vi "BotSpeak.Com.vi"(1 "To Send":string, 2 "Connection In":T1) -> (3 "error out":errorcluster, 4 "Sent":string, 5 "Reply":string, 6 "Connection out":T1)   [LabVIEW 2012]
uses:
  <userlib>/BotSpeak/VIs/SubVIs/CommState.ctl
  <userlib>/BotSpeak/VIs/Direct/BotSpeak_Control.ctl
  <userlib>/BotSpeak/VIs/SubVIs/BotSpeak_Globals.vi
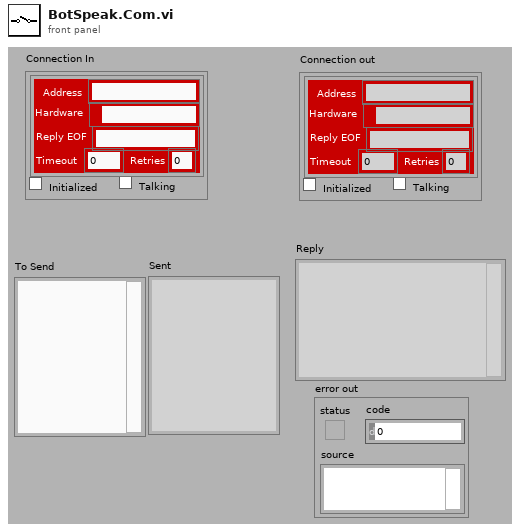
[diagram p1: front panel]
types:
  T1 = typedef "CommState.ctl" = cluster{"Bot Settings":T2, "Initialized":bool, "Talking":bool}
  T2 = typedef "BotSpeak_Control.ctl" = cluster{"Address":string, "Reply EOF":string, "Hardware":path, "Retries":i8, "Timeout":i32}
  T3 = typedef "BotSpeak.HardwareSpecs.ctl" = cluster{"Hardware Name":string, "Hardware URL":string, "ComType":enum16{"Undefined", "Serial", "TCPIP", "Console"}, "TCP Port":i32, "DefaultAddress":string, "Retries":i32, "Translate":enum16{"None", "Tiny", "URAPI"}, "MaxScriptSize":i32, "MaxVarNumber":i32, "StartupWait":i32, "Patience":i32, "Startup Patience":i32, "Hardware Help":string, "Com Protocol":string, "Translator":cluster{"BotSpeak CMD":string, "CMD out":string}[], "Init Code":string, "Variable Format":enum16{"INT", "FLOAT", "FIXED"}}
  T4 = cluster{"BotSpeak CMD":string, "CMD out":string}[]
  T5 = enum16{"Undefined", "Serial", "TCPIP", "Console"}
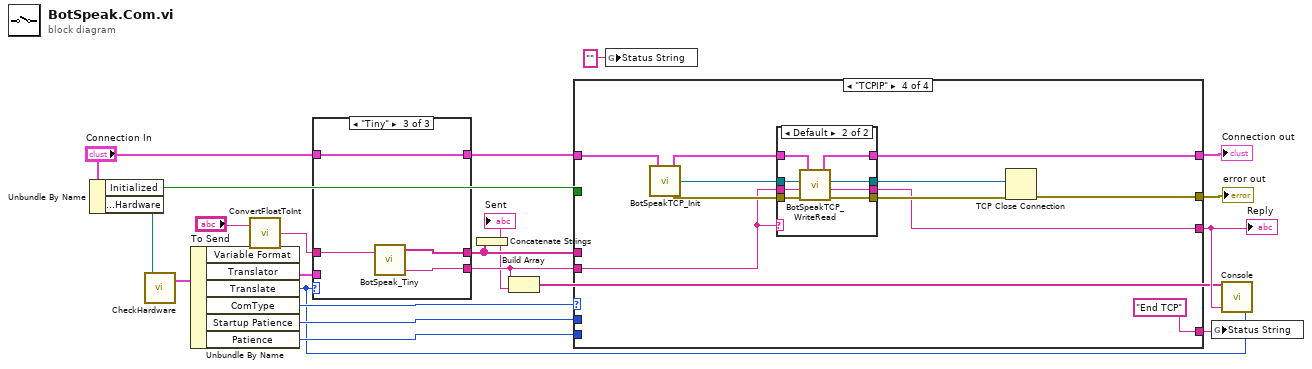
[diagram p0: block diagram]
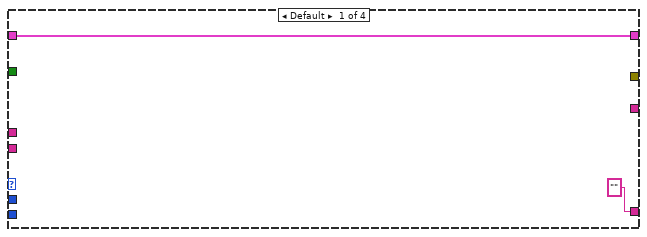
[diagram p2: hidden frame]
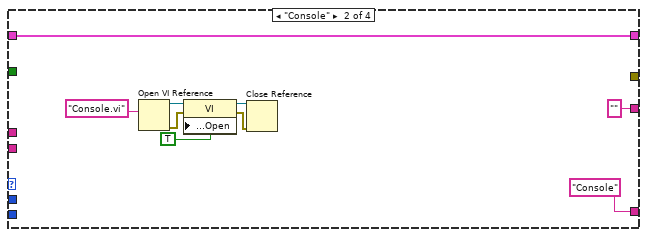
[diagram p3: hidden frame]
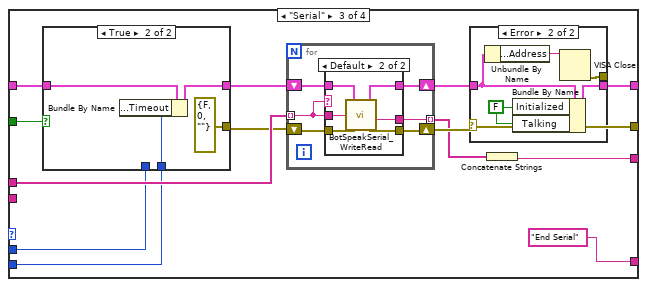
[diagram p4: hidden frame]
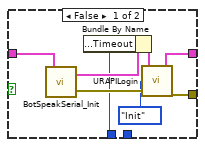
[diagram p7: hidden frame]
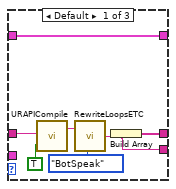
[diagram p9: hidden frame]
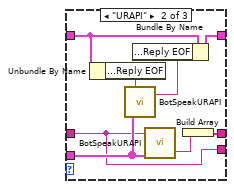
[diagram p10: hidden frame]
diagram:
  n1 = Unbundle By Name("Connection In") -> ("Initialized"=w22:bool, "Bot Settings.Hardware"=w20:path)
  n2 = call <userlib>:"CheckHardware.vi"("Hardware"=w20) -> ("HardwareSpecs"=w16:T3)  [unwired: 2 in]
  n3 = Unbundle By Name(w16) -> ("Variable Format"=w1:enum16{"INT", "FLOAT", "FIXED"}, "Translator"=w15:T4, "Translate"=w4:enum16{"None", "Tiny", "URAPI"}, "ComType"=w19:T5, "Startup Patience"=w14:i32, "Patience"=w5:i32)
  n4 = call <userlib>:"ConvertFloatToInt.vi"("Variable Format"=w1, "To Send in"="To Send") -> ("To Send out"=w2:string)
  n5 = case shown="\"Tiny\"" w4 {
    tunnel: w2 -> [w24 w30 w41]
    tunnel: [w28 w31 w40] -> w21
    tunnel: w15 -> [_ w36 _]
    tunnel: [w29 w34 w39] -> w11
    tunnel: "Connection In" -> [w29 w35 w39]
    tunnel: [w25 w30 w38] -> w9
    frame Default {
      n6 = call <userlib>:"URAPICompile.vi"("Comments?"=TRUE, "Script"=w24) -> ("trimmed script"=w26:string)
      n7 = call <userlib>:"RewriteLoopsETC.vi"("Type"=enum16{"Tiny", "BotSpeak"}."BotSpeak", "URAPI in"=w26) -> ("URAPI out"=w25:string)
      n8 = Build Array(w25) -> (w28:string[])
    }
    frame "URAPI" {
      n9 = Unbundle By Name(w35) -> ("Bot Settings.Reply EOF"=w37:string)
      n10 = call <userlib>:"BotSpeakURAPI.vi"("Translator"=w36, "To Send"=w37) -> ("translated"=w33:string)  [unwired: 1 out]
      n11 = Bundle By Name(cluster=w35, "Bot Settings.Reply EOF"=w33) -> (w34:T1)
      n12 = call <userlib>:"BotSpeakURAPI.vi"("Translator"=w36, "To Send"=w30) -> ("translated w \\n"=w32:string)  [unwired: 1 out]
      n13 = Build Array(w32) -> (w31:string[])
    }
    frame "Tiny" {
      n14 = call <userlib>:"BotSpeak_Tiny.vi"("URAPI"=w41) -> ("URAPI  2"=w38:string, "Tiny Lines"=w40:string[])  [unwired: 1 in, 1 out]
    }
  }
  n15 = Concatenate Strings(w21) -> (w8:string)
  "Sent" <- w8
  n16 = Build Array(w9, w8) -> (w6:string[])
  n17 = case shown="\"TCPIP\"" w19 {
    tunnel: w22 -> [_ _ w65 _]
    tunnel: w21 -> [_ _ w64 _]
    tunnel: [_ "" ("data out") w54 w100] -> w7
    tunnel: [_ _ w59 w102] -> w18
    tunnel: w11 -> [w43 w52 w63 w105]
    tunnel: [w43 w52 w57 w108] -> w13
    tunnel: w14 -> [_ _ w60 _]
    tunnel: ["" ("Status String") "Console" ("Status String") "End Serial" ("Status String") "End TCP" ("Status String")] -> w12
    tunnel: w9 -> [_ _ _ w99]
    tunnel: w5 -> [_ _ w53 _]
    frame Default {
    }
    frame "Console" {
      n18 = Open VI Reference(vi path="Console.vi" ("Status String")) -> (vi reference=w49:refnum<vi>, error out=w48:errorcluster)  [unwired: 5 in]
      n19 = property class="VI"(reference=w49, error in=w48, "Front Panel.Open"=TRUE ("Front Panel Window:Open")) -> (reference out=w45:refnum<vi>, error out=w46:errorcluster)
      n20 = Close Reference(reference=w45, error in (no error)=w46) -> ()  [unwired: 1 out]
    }
    frame "Serial" {
      n21 = case shown="True" w65 {
        tunnel: [w91 errorcluster {"status"=FALSE, "code"=0, "source"=""} ("error out")] -> w61
        tunnel: w63 -> [w94 w97]
        tunnel: [w92 w96] -> w62
        tunnel: w60 -> [w87 _]
        tunnel: w53 -> [_ w95]
        frame False {
          n22 = call <userlib>:"BotSpeakSerial_Init.vi"("Connection In"=w94) -> ("error out"=w93:errorcluster, "Connection out"=w89:T1)  [unwired: 1 in]
          n23 = Bundle By Name(cluster=w89, "Bot Settings.Timeout"=w87) -> (w88:T1)
          n24 = call <userlib>:"URAPILogin.vi"("error in"=w93, "Task"=enum16{"Init", "Close"}."Init", "Connection in"=w88) -> ("error out"=w91:errorcluster, "Connection Out"=w92:T1)
        }
        frame True {
          n25 = Bundle By Name(cluster=w97, "Bot Settings.Timeout"=w95) -> (w96:T1)
        }
      }
      n26 = for {
        tunnel: w64 -> [w66] mode=indexing
        tunnel: [w71] -> w55 mode=indexing
        shift-right: [w67] -> w58
        shift-left: w62 -> [w70]
        shift-right: [w68] -> w59
        shift-left: w61 -> [w69]
        n27 = case shown="Default" w66 {
          tunnel: w66 -> [w72 w80]
          tunnel: [w72 w79] -> w71
          tunnel: w70 -> [w74 w78]
          tunnel: w69 -> [w73 w77]
          tunnel: [w73 w76] -> w68
          tunnel: [w74 w75] -> w67
          frame "" {
          }
          frame Default {
            n28 = call <userlib>:"BotSpeakSerial_WriteRead.vi"("error In"=w77, "To Write"=w80, "Connection In"=w78) -> ("error out"=w76:errorcluster, "Reply"=w79:string, "Connection Out"=w75:T1)  [unwired: 1 out]
          }
        }
      }
      n29 = case shown="Error" w59 {
        tunnel: [w81 w86] -> w57
        tunnel: w58 -> [w81 w84]
        tunnel: [_ w82] -> _
        frame No Error {
        }
        frame Error {
          w85 = FALSE ("Initialized")
          n30 = Unbundle By Name(w84) -> ("Bot Settings.Address"=w83:string)
          n31 = Bundle By Name(cluster=w84, "Initialized"=w85, "Talking"=w85) -> (w86:T1)
          n32 = VISA Close(VISA resource name=w83) -> (error out=w82:errorcluster)  [unwired: 1 in]
        }
      }
      n33 = Concatenate Strings(w55) -> (w54:string)
    }
    frame "TCPIP" {
      n34 = call <userlib>:"BotSpeakTCP_Init.vi"("Connection In"=w105) -> ("error out"=w106:errorcluster, "connection ID"=w107:refnum<k5>, "Connection Out"=w109:T1)  [unwired: 1 in]
      n35 = case shown="Default" w99 {
        tunnel: w109 -> [w113 w121]
        tunnel: [w113 w120] -> w108
        tunnel: w107 -> [w112 w119]
        tunnel: w106 -> [w110 w118]
        tunnel: [w112 w117] -> w104
        tunnel: [w110 w116] -> w103
        tunnel: [w111 w115] -> w100
        tunnel: w99 -> [w111 w114]
        frame "" {
        }
        frame Default {
          n36 = call <userlib>:"BotSpeakTCP_WriteRead.vi"("error in"=w118, "To Send"=w114, "connection ID"=w119, "Connection In"=w121) -> ("error out"=w116:errorcluster, "data out"=w115:string, "connection ID out"=w117:refnum<k5>, "Connection Out"=w120:T1)
        }
      }
      n37 = TCP Close Connection(connection ID=w104, error in (no error)=w103) -> (error out=w102:errorcluster)  [unwired: 1 in, 1 out]
    }
  }
  "Reply" <- w7
  "error out" <- w18
  "Connection out" <- w13
  n38 = global write "BotSpeak_Globals.vi" "Status String"("" ("Status String")) -> ()
  n39 = global write "BotSpeak_Globals.vi" "Status String"(w12) -> ()
  n40 = call <userlib>:"Console.vi"("Translate"=w4, "Reply"=w7, "Sent"=w6) -> ()  [unwired: 1 in, 2 out]
